vi "ColorLimits.vi"(8 "error in":errorcluster, 9 "ctlRef_Limits":refnum<vi>[](array[refnum]), 11 "PredictiveMaintenance in":refnum<class "PredictiveMaintenance.lvclass">) -> (0 "error out":errorcluster, 3 "PredictiveMaintenance OUT":refnum<class "PredictiveMaintenance.lvclass">)   [LabVIEW 2019, in "PredictiveMaintenance.lvlib" / "PredictiveMaintenance.lvclass"]
uses:
  PredictiveMaintenance.lvclass
  PredictiveMaintenance.lvclass/PredictiveMaintenance.ctl
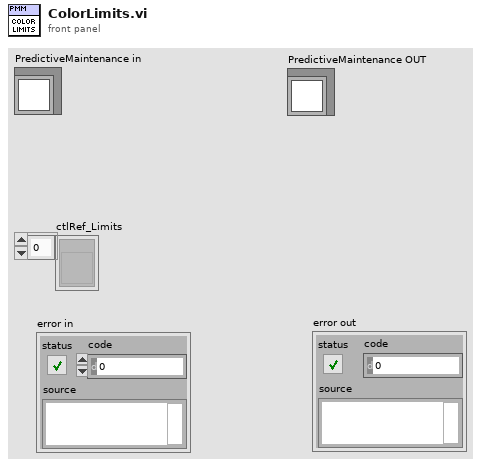
[diagram p1: front panel]
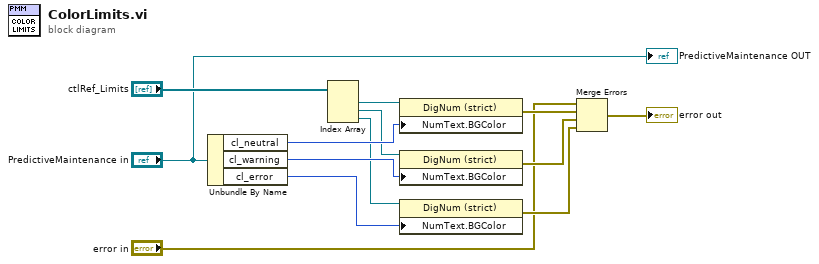
[diagram p0: block diagram]
diagram:
  n1 = Unbundle By Name("PredictiveMaintenance in") -> ("cl_neutral"=w11:u32, "cl_warning"=w12:u32, "cl_error"=w13:u32)
  n2 = Index Array(array="ctlRef_Limits") -> (element #1=w10:refnum<vi>, element #2=w9:refnum<vi>, element #3=w8:refnum<vi>)  [unwired: 3 in]
  n3 = property class="DigNum (strict)"(reference=w10, "NumText.BGColor"=w11) -> (error out=w7:errorcluster)  [unwired: 1 in, 1 out]
  n4 = property class="DigNum (strict)"(reference=w9, "NumText.BGColor"=w12) -> (error out=w6:errorcluster)  [unwired: 1 in, 1 out]
  n5 = property class="DigNum (strict)"(reference=w8, "NumText.BGColor"=w13) -> (error out=w5:errorcluster)  [unwired: 1 in, 1 out]
  n6 = Merge Errors("error in", w7, w6, w5) -> (→"error out":errorcluster)
  "PredictiveMaintenance OUT" <- "PredictiveMaintenance in"
